vi "W Station Strings.vi"(8 "Length":i32=12, 9 "Starting Number":i32, 11 "Station Prefix Letter":string="W") -> (3 "W Array":string[](array[string]))   [LabVIEW 2009]
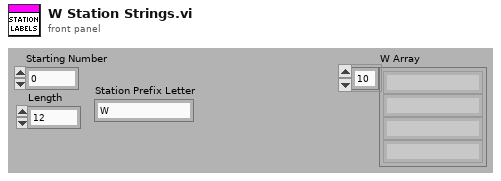
[diagram p1: front panel]
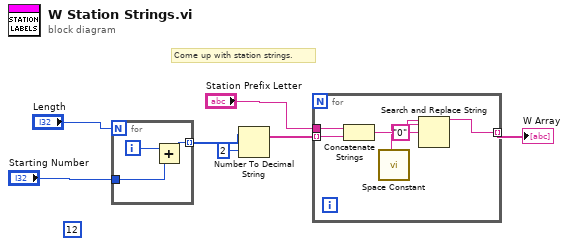
[diagram p0: block diagram]
diagram:
  (unwired) 12
  # "Come up with station strings."
  n1 = for {
    N: "Length" -> [_]
    tunnel: [w9] -> w6 mode=indexing
    tunnel: "Starting Number" -> [w8]
    i -> [w10]
    n2 = Add(x=w10, y=w8) -> (x+y=w9:i32)
  }
  n3 = Number To Decimal String(number=w6, width (-)=i16 2) -> (decimal integer string=w4:string[])
  n4 = for {
    tunnel: w4 -> [w16] mode=indexing
    tunnel: "Station Prefix Letter" -> [w15]
    tunnel: [w14] -> w2 mode=indexing
    n5 = Concatenate Strings(w15, w16) -> (w13:string)
    n6 = call <vilib>:"Space Constant.vi"() -> ("String"=w12:string)
    n7 = Search and Replace String(input string=w13, search string=w12, replace string="0" ("replace string (\"\")")) -> (result string=w14:string)  [unwired: 5 in, 3 out]
  }
  "W Array" <- w2
